vi "merFISH_path_definition.vi"(3 "error in":errorcluster, 4 "Sample name":string="RAMM_Test", 5 "Saving path":path=path "E:/") -> (0 "error out":errorcluster, 1 "Saving path":path, 2 "merFISH path":path)   [LabVIEW 2015]
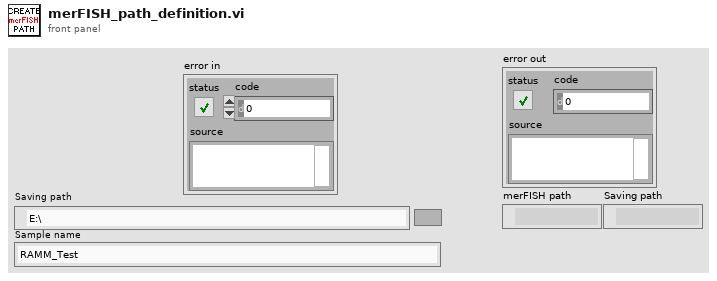
[diagram p1: front panel]
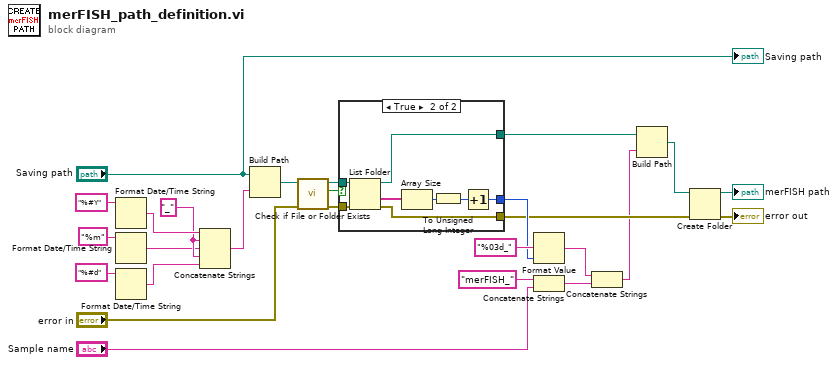
[diagram p0: block diagram]
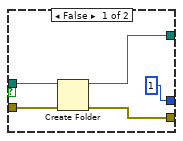
[diagram p2: hidden frame]
diagram:
  w24 = "_" ("string")
  n1 = Format Date/Time String(time format string (%c)="%#Y") -> (date/time string=w25:string)  [unwired: 2 in]
  n2 = Format Date/Time String(time format string (%c)="%m") -> (date/time string=w21:string)  [unwired: 2 in]
  n3 = Format Date/Time String(time format string (%c)="%#d") -> (date/time string=w20:string)  [unwired: 2 in]
  n4 = Concatenate Strings(w25, w24, w21, w24, w20) -> (w19:string)
  n5 = Build Path(base path="Saving path", name or relative path=w19) -> (appended path=w18:path)
  n6 = call <vilib>:"Check if File or Folder Exists.vi"("error in (no error)"="error in", "path"=w18) -> ("error out"=w16:errorcluster, "file or folder exists?"=w17:bool, "dup path"=w15:path)  [unwired: 7 in]
  n7 = case shown="True" w17 {
    tunnel: w16 -> [w31 w38]
    tunnel: [w28 w34] -> w8
    tunnel: w15 -> [w30 w39]
    tunnel: [w29 w35] -> w14
    tunnel: [u32 1 w33] -> w9
    frame False {
      n8 = Create Folder(path (use dialog)=w30, error in=w31) -> (created path=w29:path, error out=w28:errorcluster)  [unwired: 1 in, 1 out]
    }
    frame True {
      n9 = List Folder(path=w39, error in=w38) -> (path out=w35:path, folder names=w36:string[], error out=w34:errorcluster)  [unwired: 2 in, 1 out]
      n10 = Array Size(array=w36) -> (size(s)=w37:i32)
      n11 = To Unsigned Long Integer(number=w37) -> (unsigned 32bit integer=w32:u32)
      n12 = Increment(x=w32) -> (x+1=w33:u32)
    }
  }
  n13 = Format Value(format string="%03d_" ("string (\"\")"), value (0)=w9) -> (output string=w11:string)  [unwired: 1 in]
  n14 = Concatenate Strings("merFISH_" ("string"), "Sample name") -> (w10:string)
  n15 = Concatenate Strings(w11, w10) -> (w7:string)
  n16 = Build Path(base path=w14, name or relative path=w7) -> (appended path=w6:path)
  n17 = Create Folder(path (use dialog)=w6, error in=w8) -> (created path=→"merFISH path":path, error out=→"error out":errorcluster)  [unwired: 1 in, 1 out]
  "Saving path" <- "Saving path"
